vi "TPS Global.vi"() -> ()   [LabVIEW 2019]
doc: "This Global is written to by TPS System Start."
panel:
  in  "TPS Setup File":string="B28_Setup_File.txt"
  in  "TPS Base Path":path=path "C:/Users/ptgroup/Documents/PDP"
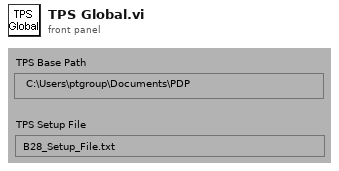
[diagram p1: front panel]
diagram:
